vi "Flow Rate Sensor Range--constant.vi"() -> (2 "Min":dbl, 3 "Max":dbl=50.0)   [LabVIEW 2024, in "Hardware Controller.lvlib"]
uses:
  Hardware Controller.lvlib
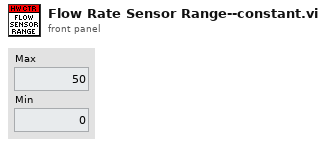
[diagram p1: front panel]
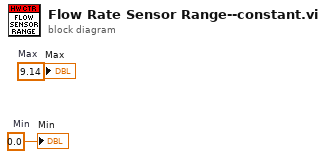
[diagram p0: block diagram]
diagram:
  w1 = 0.0  # Min
  w2 = 9.14  # Max
  "Max" <- w2
  "Min" <- w1
